vi "Write Speaker_.vi"(8 "error in (no error)":errorcluster, 10 "Speaker?":bool, 11 "Change Speaker Switch in":refnum<class "Change Speaker Switch MSG.lvclass">) -> (0 "error out":errorcluster, 3 "Change Speaker Switch out":refnum<class "Change Speaker Switch MSG.lvclass">)   [LabVIEW 2014, in "ePAS Library.lvlib" / "Change Speaker Switch MSG.lvclass"]
uses:
  Change Speaker Switch MSG.lvclass
  Change Speaker Switch MSG.lvclass/Change Speaker Switch MSG.ctl
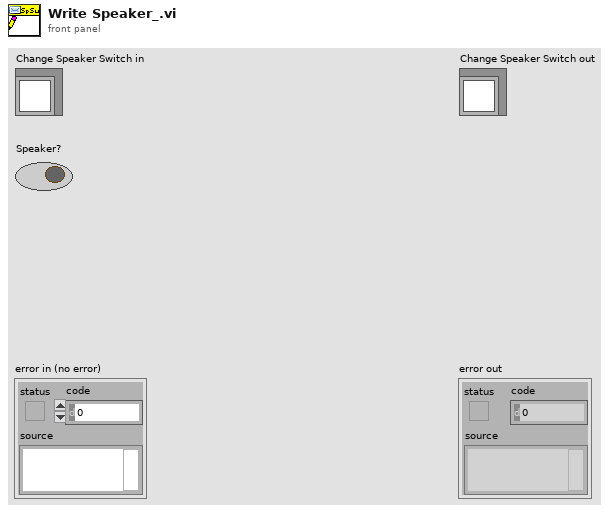
[diagram p1: front panel]
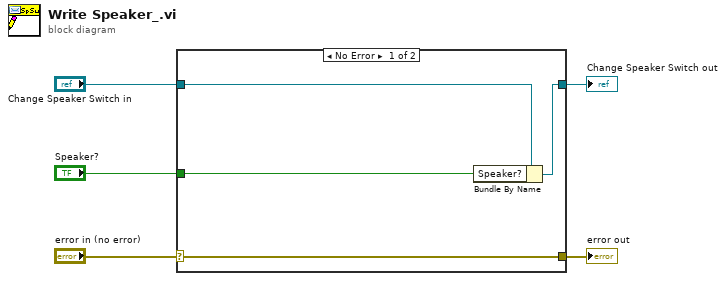
[diagram p0: block diagram]
diagram:
  n1 = case shown="No Error" "error in (no error)" {
    selector: "error in (no error)" -> [w9 w10]
    tunnel: [w9 w10] -> w4
    tunnel: [w7 w11] -> w2
    tunnel: "Change Speaker Switch in" -> [w8 w11]
    tunnel: "Speaker?" -> [w6 _]
    frame No Error {
      n2 = Bundle By Name(cluster=w8, "Speaker?"=w6) -> (w7:refnum<class "Change Speaker Switch MSG.lvclass">)
    }
    frame Error {
    }
  }
  "error out" <- w4
  "Change Speaker Switch out" <- w2
